vi "fgv_logbuff_q.vi"(7 "cmd":T1, 8 "error in":errorcluster, 11 "data":string) -> (0 "error out":errorcluster, 3 "queue out":refnum<queue>)   [LabVIEW 2019]
uses:
  Ctrl/log_buffq.ctl
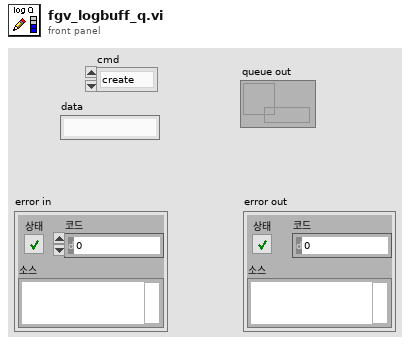
[diagram p1: front panel]
types:
  T1 = typedef "log_buffq.ctl" = enum16{"create", "write", "read", "close"}
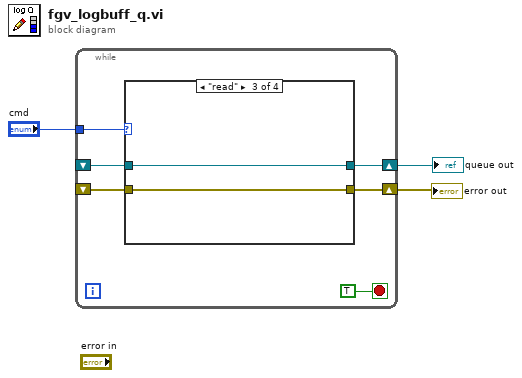
[diagram p0: block diagram]
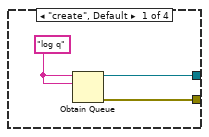
[diagram p2: hidden frame]
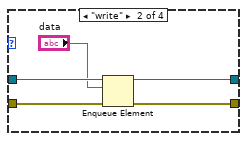
[diagram p3: hidden frame]
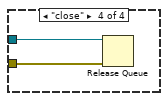
[diagram p4: hidden frame]
diagram:
  n1 = while {
    tunnel: "cmd" -> [w8]
    shift-right: [w7] -> w2
    shift-left: _ -> [w4]
    shift-right: [w6] -> w1
    shift-left: _ -> [w5]
    stop <- TRUE stop-if-true
    n2 = case shown="\"read\"" w8 {
      tunnel: [w11 w15 w19 _] -> w7
      tunnel: [w10 w16 w18 _] -> w6
      tunnel: w5 -> [_ w17 w18 w21]
      tunnel: w4 -> [_ w14 w19 w20]
      frame "create", Default {
        w12 = "log q" ("이름(이름없음)")
        n3 = Obtain Queue(name (unnamed)=w12, element data type=w12) -> (queue out=w11:refnum<queue>, error out=w10:errorcluster)  [unwired: 3 in, 1 out]
      }
      frame "write" {
        n4 = Enqueue Element(queue=w14, element="data", error in (no error)=w17) -> (queue out=w15:refnum<queue>, error out=w16:errorcluster)  [unwired: 1 in, 1 out]
      }
      frame "read" {
      }
      frame "close" {
        n5 = Release Queue(queue=w20, error in (no error)=w21) -> ()  [unwired: 1 in, 3 out]
      }
    }
  }
  "queue out" <- w2
  "error out" <- w1
